vi "Write Writer Class.vi"(2 "EnclaveChannel":T1) -> (7 "Writer":refnum<class "Writer.lvclass">)   [LabVIEW 2022 SP3, in "Enclave.lvlib"]
doc: "Creates a class instance that enables writing values to connected readers."
uses:
  Enclave.lvlib
  ))Channel.ctl
  Element.ctl
  Writer/Writer.lvclass
  Operation.ctl
  Enclave/Enclave.lvclass
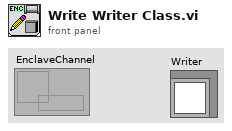
[diagram p1: front panel]
types:
  T1 = typedef "Enclave.lvlib/))Channel.ctl" = refnum<queue>
  T2 = typedef "Enclave.lvlib/Operation.ctl" = enum16{"Get Core", "Init", "Close"}
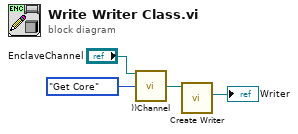
[diagram p0: block diagram]
diagram:
  n1 = call "))Channel.vi"("EnclaveChannel in"="EnclaveChannel", "Operation"=Operation."Get Core") -> ("Enclave"=w2:refnum<class "Enclave.lvclass">)  [unwired: 11 in, 2 out]
  n2 = call "Create Writer.vi"("Enclave in"=w2) -> ("Writer"=→"Writer":refnum<class "Writer.lvclass">)  [unwired: 8 in, 2 out]
